vi "插入模式.vi"(8 "模式":T2, 11 "模式列表":T1(array[cluster])) -> (3 "模式列表-output":T1(array[cluster]))   [LabVIEW 2019]
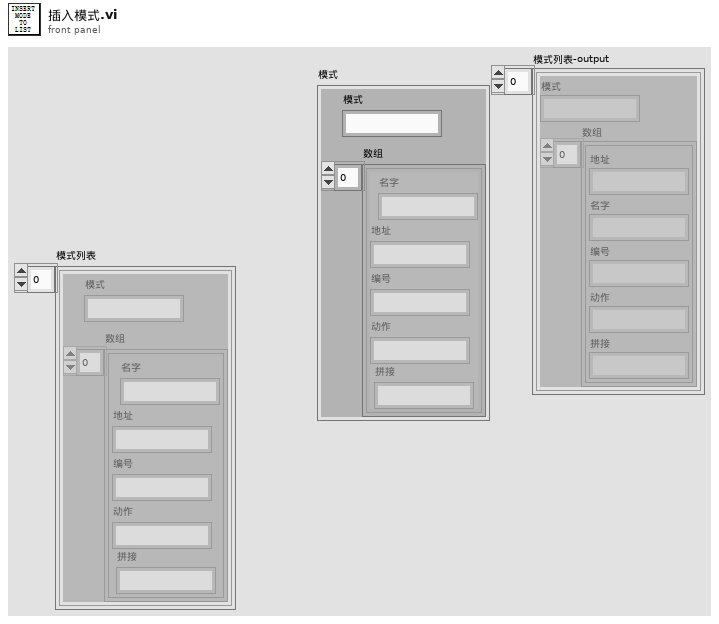
[diagram p1: front panel]
types:
  T1 = cluster{"模式":string, "数组":cluster{"地址":string, "名字":string, "编号":string, "动作":string, "拼接":string}[]}[]
  T2 = cluster{"模式":string, "数组":cluster{"地址":string, "名字":string, "编号":string, "动作":string, "拼接":string}[]}
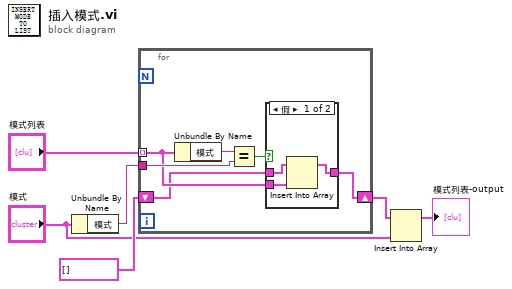
[diagram p0: block diagram]
diagram:
  n1 = Unbundle By Name("模式") -> ("模式"=w5:string)
  n2 = for {
    tunnel: "模式列表" -> [w8] mode=indexing
    shift-right: [w9] -> w3
    shift-left: T1 [] -> [w7]
    tunnel: w5 -> [w11]
    n3 = Unbundle By Name(w8) -> ("模式"=w12:string)
    n4 = Equal?(x=w12, y=w11) -> (x = y?=w10:bool)
    n5 = case shown="假" w10 {
      tunnel: [w15 w16] -> w9
      tunnel: w8 -> [w14 _]
      tunnel: w7 -> [w13 w16]
      frame False {
        n6 = Insert Into Array(array=w13, new element=w14) -> (w15:T1)  [unwired: 1 in]
      }
      frame True {
      }
    }
  }
  n7 = Insert Into Array(array=w3, new element="模式") -> (→"模式列表-output":T1)  [unwired: 1 in]
